vi "XYZ stage communication_MD.vi"   [LabVIEW 2012]
uses:
  <vilib>/Utility/VariantDataType/Type.ctl
  GFG/GFGstringGet.vi
  <vilib>/Instr/_visa.llb/VISA Configure Serial Port (Instr).vi
  GFG/GFGnumericGet.vi
  GFG/GFGbooleanGet.vi
  GFG/GFG library.lvlib
  <vilib>/Utility/VariantDataType/VariantType.lvlib
types:
  T1 = cluster{"moveXabs":dbl, "moveYabs":dbl, "moveZabs":dbl}
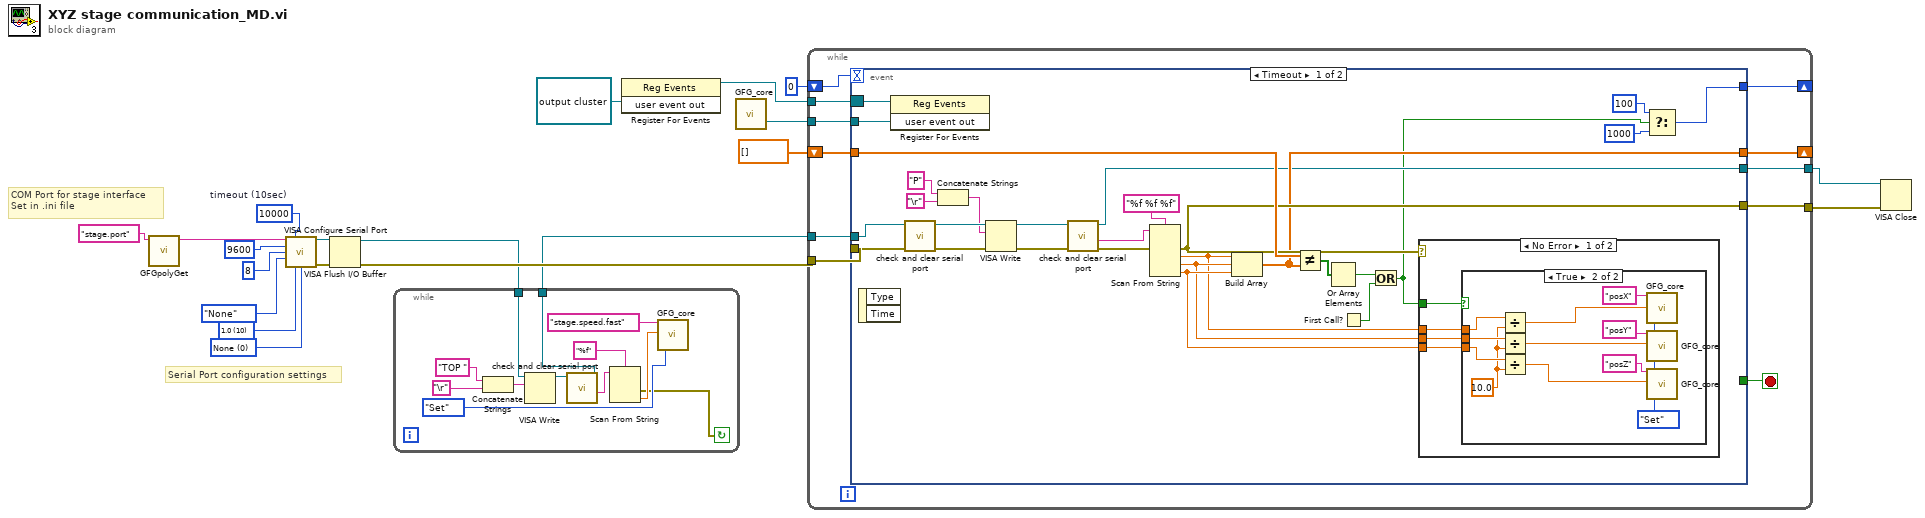
[diagram p0: block diagram]
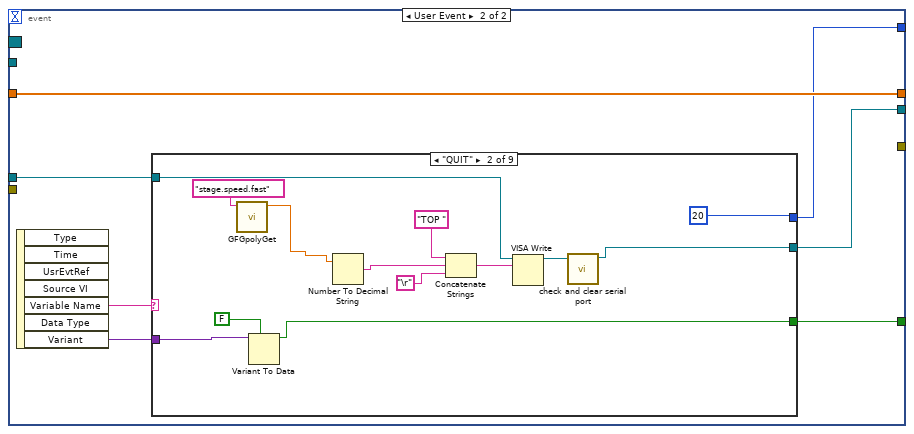
[diagram p4: hidden frame]
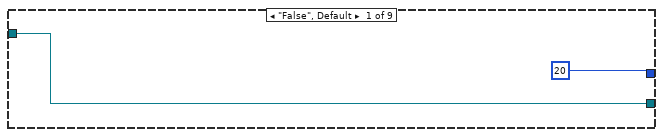
[diagram p5: hidden frame]
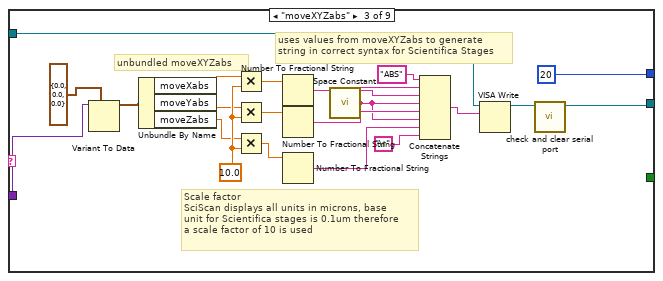
[diagram p6: hidden frame]
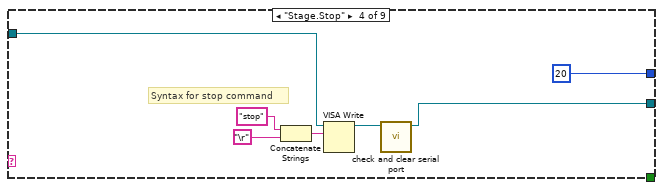
[diagram p7: hidden frame]
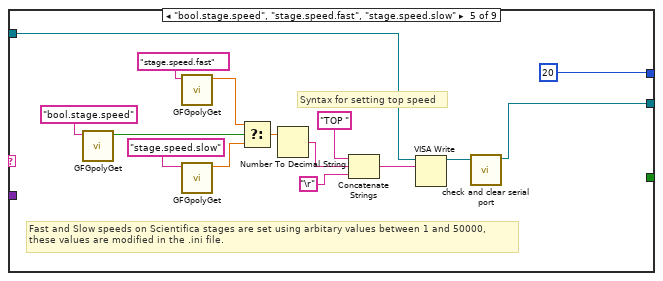
[diagram p8: hidden frame]
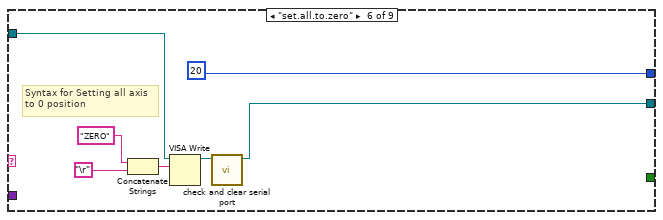
[diagram p9: hidden frame]
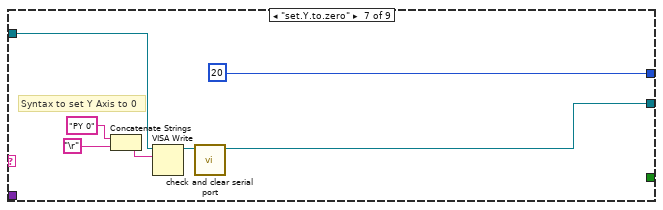
[diagram p10: hidden frame]
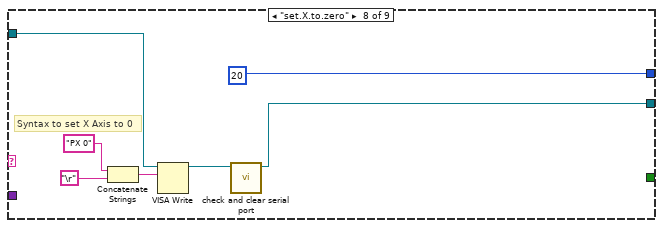
[diagram p11: hidden frame]
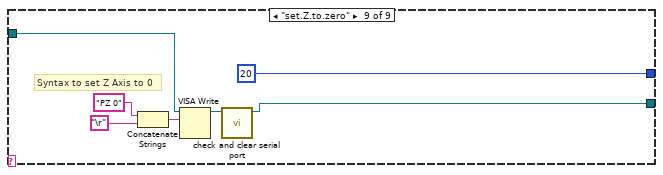
[diagram p12: hidden frame]
diagram:
  w13 = u16 0 items=["None", "XON/XOFF", "RTS/CTS", "XON/XOFF & RTS/CTS", "DTR/DSR", "XON/XOFF & DTR/DSR"] ("flow control (0:none)")
  w14 = u16 10 items=["1.0"=10, "1.5"=15, "2.0"=20] ("stop bits (10: 1 bit)")
  w18 = u32 10000  # timeout (10sec)
  # "COM Port for stage interface\nSet in .ini file"
  # "Serial Port configuration settings"
  n1 = call-poly "GFGpolyGet.vi"("Variable Name in"="stage.port") -> ("String"=w10:string)  [unwired: 10 in]
  n2 = call-poly "VISA Configure Serial Port"("VISA resource name"=w10, "timeout (10sec)"=w18, "baud rate (9600)"=u32 9600, "data bits (8)"=u16 8, "parity (0:none)"=enum16{"None", "Odd", "Even", "Mark", "Space"}."None", "stop bits (10: 1 bit)"=w14, "flow control (0:none)"=w13) -> ("VISA resource name out"=w12:refnum<visa-resource-name>, "error out"=w11:errorcluster)  [unwired: 7 in]
  n3 = VISA Flush I/O Buffer(VISA resource name=w12, error in (no error)=w11) -> (VISA resource name out=w2:refnum<visa-resource-name>, error out=w7:errorcluster)  [unwired: 1 in]
  n4 = while {
    tunnel: w2 -> [w28]
    tunnel: [w27] -> w1
    stop <- w21 continue-if-true
    n5 = Concatenate Strings("TOP " ("write buffer"), "\r") -> (w31:string)
    n6 = VISA Write(VISA resource name=w28, write buffer=w31) -> (VISA resource name out=w30:refnum<visa-resource-name>)  [unwired: 1 in, 2 out]
    n7 = call "check and clear serial port.vi"("VISA resource name in"=w30) -> ("read buffer"=w23:string, "VISA resource name out"=w27:refnum<visa-resource-name>)  [unwired: 7 in, 2 out]
    n8 = Scan From String(format string="%f", input string=w23) -> (error out=w21:errorcluster, output 1=w22:dbl)  [unwired: 3 in, 2 out]
    n9 = call "GFG_core.vi"("Variable Name in"="stage.speed.fast", "Variant in"=w22, "Action"=enum16{"Init", "Set", "Get"}."Set") -> ()  [unwired: 10 in, 7 out]
  }
  n10 = register-events(refnum<user-event> refnum ("user event out")) -> (reference out=w3:refnum<event-registration>)  [unwired: 2 in, 1 out]
  n11 = call "GFG_core.vi"() -> ("user event out"=w8:refnum<user-event>)  [unwired: 13 in, 6 out]
  n12 = while {
    tunnel: [w43] -> w6
    tunnel: w1 -> [w42]
    shift-right: [w41] -> _
    shift-left: dbl[] [] -> [w39]
    tunnel: w7 -> [w38]
    tunnel: [w37] -> w5
    shift-right: [w35] -> _
    shift-left: 0 -> [w36]
    tunnel: w8 -> [w34]
    tunnel: w3 -> [w33]
    stop <- w40 stop-if-true
    n13 = event shown="[0] Timeout" {
      selector: w33 -> [w48 _]
      dyn-events: _ -> [_ _]
      timeout: w36 -> [_ _]
      tunnel: [w57 w89] -> w43
      tunnel: w42 -> [w66 w90]
      tunnel: [w69 w88] -> w41
      tunnel: [_ w91] -> w40
      tunnel: w39 -> [w71 w88]
      tunnel: w38 -> [w64 _]
      tunnel: [w70 _] -> w37
      tunnel: [w51 w87] -> w35
      tunnel: w34 -> [w47 _]
      event Timeout {
        n14 = event-data() -> ()  [unwired: 1 in, 2 out]
        n15 = register-events(reference=w48, w47) -> ()  [unwired: 1 in, 2 out]
        n16 = call "check and clear serial port.vi"("error in (no error)"=w64, "VISA resource name in"=w66) -> ("error out"=w63:errorcluster, "VISA resource name out"=w65:refnum<visa-resource-name>)  [unwired: 6 in, 2 out]
        n17 = Concatenate Strings("P" ("write buffer"), "\r") -> (w55:string)
        n18 = VISA Write(VISA resource name=w65, write buffer=w55, error in (no error)=w63) -> (VISA resource name out=w59:refnum<visa-resource-name>, error out=w60:errorcluster)  [unwired: 1 out]
        n19 = call "check and clear serial port.vi"("error in (no error)"=w60, "VISA resource name in"=w59) -> ("error out"=w58:errorcluster, "read buffer"=w56:string, "VISA resource name out"=w57:refnum<visa-resource-name>)  [unwired: 6 in, 1 out]
        n20 = Scan From String(format string="%f %f %f", input string=w56, error in=w58) -> (error out=w70:errorcluster, output 1=w44:dbl, output 2=w45:dbl, output 3=w46:dbl)  [unwired: 4 in, 2 out]
        n21 = Build Array(w44, w45, w46) -> (w69:dbl[])
        n22 = Not Equal?(x=w71, y=w69) -> (x != y?=w68:bool[])
        n23 = Or Array Elements(Boolean array=w68) -> (logical OR=w52:bool)
        n24 = First Call?() -> (First Call?: T/F=w50:bool)
        n25 = Or(x=w52, y=w50) -> (x .or. y?=w49:bool)
        n26 = case shown="No Error" w70 {
          tunnel: w44 -> [w73 _]
          tunnel: w45 -> [w74 _]
          tunnel: w46 -> [w75 _]
          tunnel: w49 -> [w72 _]
          frame No Error {
            n27 = case shown="True" w72 {
              tunnel: w75 -> [_ w83]
              tunnel: w74 -> [_ w81]
              tunnel: w73 -> [_ w79]
              frame False {
              }
              frame True {
                w78 = 10.0 ("y")
                w76 = enum16{"Init", "Set", "Get"}."Set" ("Action")
                n28 = Divide(x=w79, y=w78) -> (x/y=w77:dbl)
                n29 = Divide(x=w81, y=w78) -> (x/y=w80:dbl)
                n30 = Divide(x=w83, y=w78) -> (x/y=w82:dbl)
                n31 = call "GFG_core.vi"("Variable Name in"="posX", "Variant in"=w77, "Action"=w76) -> ()  [unwired: 10 in, 7 out]
                n32 = call "GFG_core.vi"("Variable Name in"="posY", "Variant in"=w80, "Action"=w76) -> ()  [unwired: 10 in, 7 out]
                n33 = call "GFG_core.vi"("Variable Name in"="posZ", "Variant in"=w82, "Action"=w76) -> ()  [unwired: 10 in, 7 out]
              }
            }
          }
          frame Error {
          }
        }
        n34 = Select(t=100, s=w49, f=1000) -> (s? t:f=w51:i32)
      }
      event User Event {
        n35 = event-data() -> ("Variable Name"=w93:string, "Variant"=w92:variant)  [unwired: 1 in, 5 out]
        n36 = case shown="\"QUIT\"" w93 {
          tunnel: [_ w106 _ _ _ _ _ _ _] -> w91
          tunnel: w92 -> [_ w108 w114 _ _ _ _ _ _]
          tunnel: w90 -> [w95 w101 w124 w132 w139 w156 w163 w170 w179]
          tunnel: [w95 w100 w117 w131 w138 w154 w161 w168 w178] -> w89
          tunnel: [20 20 20 20 20 20 20 20 20] -> w87
          frame "False", Default {
          }
          frame "QUIT" {
            n37 = call-poly "GFGpolyGet.vi"("Variable Name in"="stage.speed.fast") -> ("Numeric"=w98:dbl)  [unwired: 9 in, 1 out]
            n38 = Variant To Data(type=FALSE ("NewVal"), Variant=w108) -> (data=w106:bool)  [unwired: 1 in, 1 out]
            n39 = Number To Decimal String(number=w98) -> (decimal integer string=w96:string)  [unwired: 1 in]
            n40 = Concatenate Strings("TOP " ("write buffer"), w96, "\r") -> (w103:string)
            n41 = VISA Write(VISA resource name=w101, write buffer=w103) -> (VISA resource name out=w104:refnum<visa-resource-name>)  [unwired: 1 in, 2 out]
            n42 = call "check and clear serial port.vi"("VISA resource name in"=w104) -> ("VISA resource name out"=w100:refnum<visa-resource-name>)  [unwired: 7 in, 3 out]
          }
          frame "moveXYZabs" {
            w119 = 10.0 ("y")
            # "Scale factor \nSciScan displays all units in microns, base \nunit for Scientifica stages is 0.1um therefore \na scale factor of 10 is used"
            # "unbundled moveXYZabs"
            # "uses values from moveXYZabs to generate\nstring in correct syntax for Scientifica Stages"
            n43 = Variant To Data(type=T1 {"moveXabs"=0.0, "moveYabs"=0.0, "moveZabs"=0.0} ("output cluster"), Variant=w114) -> (data=w112:T1)  [unwired: 1 in, 1 out]
            n44 = Unbundle By Name(w112) -> ("moveXabs"=w109:dbl, "moveYabs"=w110:dbl, "moveZabs"=w111:dbl)
            n45 = Multiply(x=w109, y=w119) -> (x*y=w122:dbl)
            n46 = Multiply(x=w110, y=w119) -> (x*y=w121:dbl)
            n47 = Multiply(x=w111, y=w119) -> (x*y=w120:dbl)
            n48 = Number To Fractional String(number=w122) -> (F-format string=w129:string)  [unwired: 3 in]
            n49 = Number To Fractional String(number=w121) -> (F-format string=w128:string)  [unwired: 3 in]
            n50 = Number To Fractional String(number=w120) -> (F-format string=w127:string)  [unwired: 3 in]
            n51 = call <vilib>:"Space Constant.vi"() -> ("String"=w126:string)
            n52 = Concatenate Strings("ABS" ("string"), w126, w129, w126, w128, w126, w127, "\r") -> (w116:string)
            n53 = VISA Write(VISA resource name=w124, write buffer=w116) -> (VISA resource name out=w118:refnum<visa-resource-name>)  [unwired: 1 in, 2 out]
            n54 = call "check and clear serial port.vi"("VISA resource name in"=w118) -> ("VISA resource name out"=w117:refnum<visa-resource-name>)  [unwired: 7 in, 3 out]
          }
          frame "Stage.Stop" {
            # "Syntax for stop command"
            n55 = Concatenate Strings("stop" ("write buffer"), "\r") -> (w136:string)
            n56 = VISA Write(VISA resource name=w132, write buffer=w136) -> (VISA resource name out=w135:refnum<visa-resource-name>)  [unwired: 1 in, 2 out]
            n57 = call "check and clear serial port.vi"("VISA resource name in"=w135) -> ("VISA resource name out"=w131:refnum<visa-resource-name>)  [unwired: 7 in, 3 out]
          }
          frame "bool.stage.speed", "stage.speed.fast", "stage.speed.slow" {
            # "Syntax for setting top speed"
            # "Fast and Slow speeds on Scientifica stages are set using arbitary values between 1 and 50000, \nthese values are modified in the .ini file."
            n58 = call-poly "GFGpolyGet.vi"("Variable Name in"="bool.stage.speed") -> ("Boolean"=w142:bool)  [unwired: 10 in]
            n59 = call-poly "GFGpolyGet.vi"("Variable Name in"="stage.speed.fast") -> ("Numeric"=w144:dbl)  [unwired: 9 in, 1 out]
            n60 = call-poly "GFGpolyGet.vi"("Variable Name in"="stage.speed.slow") -> ("Numeric"=w143:dbl)  [unwired: 9 in, 1 out]
            n61 = Select(t=w144, s=w142, f=w143) -> (s? t:f=w141:dbl)
            n62 = Number To Decimal String(number=w141) -> (decimal integer string=w140:string)  [unwired: 1 in]
            n63 = Concatenate Strings("TOP " ("write buffer"), w140, "\r") -> (w150:string)
            n64 = VISA Write(VISA resource name=w139, write buffer=w150) -> (VISA resource name out=w151:refnum<visa-resource-name>)  [unwired: 1 in, 2 out]
            n65 = call "check and clear serial port.vi"("VISA resource name in"=w151) -> ("VISA resource name out"=w138:refnum<visa-resource-name>)  [unwired: 7 in, 3 out]
          }
          frame "set.all.to.zero" {
            # "Syntax for Setting all axis \nto 0 position"
            n66 = Concatenate Strings("ZERO" ("write buffer"), "\r") -> (w152:string)
            n67 = VISA Write(VISA resource name=w156, write buffer=w152) -> (VISA resource name out=w155:refnum<visa-resource-name>)  [unwired: 1 in, 2 out]
            n68 = call "check and clear serial port.vi"("VISA resource name in"=w155) -> ("VISA resource name out"=w154:refnum<visa-resource-name>)  [unwired: 7 in, 3 out]
          }
          frame "set.Y.to.zero" {
            # "Syntax to set Y Axis to 0"
            n69 = Concatenate Strings("PY 0" ("write buffer"), "\r") -> (w160:string)
            n70 = VISA Write(VISA resource name=w163, write buffer=w160) -> (VISA resource name out=w162:refnum<visa-resource-name>)  [unwired: 1 in, 2 out]
            n71 = call "check and clear serial port.vi"("VISA resource name in"=w162) -> ("VISA resource name out"=w161:refnum<visa-resource-name>)  [unwired: 7 in, 3 out]
          }
          frame "set.X.to.zero" {
            # "Syntax to set X Axis to 0"
            n72 = Concatenate Strings("PX 0" ("write buffer"), "\r") -> (w167:string)
            n73 = VISA Write(VISA resource name=w170, write buffer=w167) -> (VISA resource name out=w169:refnum<visa-resource-name>)  [unwired: 1 in, 2 out]
            n74 = call "check and clear serial port.vi"("VISA resource name in"=w169) -> ("VISA resource name out"=w168:refnum<visa-resource-name>)  [unwired: 7 in, 3 out]
          }
          frame "set.Z.to.zero" {
            # "Syntax to set Z Axis to 0"
            n75 = Concatenate Strings("PZ 0" ("write buffer"), "\r") -> (w173:string)
            n76 = VISA Write(VISA resource name=w179, write buffer=w173) -> (VISA resource name out=w174:refnum<visa-resource-name>)  [unwired: 1 in, 2 out]
            n77 = call "check and clear serial port.vi"("VISA resource name in"=w174) -> ("VISA resource name out"=w178:refnum<visa-resource-name>)  [unwired: 7 in, 3 out]
          }
        }
      }
    }
  }
  n78 = VISA Close(VISA resource name=w6, error in (no error)=w5) -> ()  [unwired: 1 out]
